vi "GVMetavariablen.vi"() -> ()   [LabVIEW 2010]
panel:
  out "MVFix?":bool[](array[boolean])
  in  "MVFixwert":dbl[](array[numeric])
  out "Metavariablen":dbl[](array[numeric])
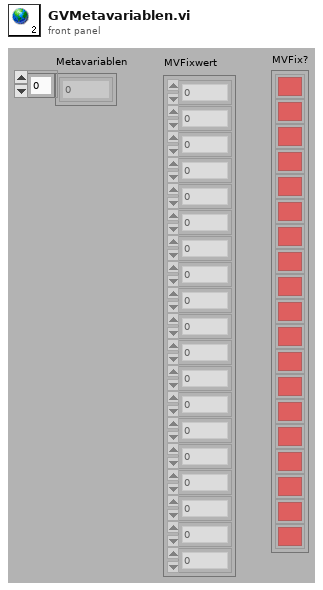
[diagram p1: front panel]
diagram:
